vi "Control_DAQ.vi"(7 "Transfer Function":T5={"Transfer Function"={"Numerator"=[1.0], "Denominator"=[-0.9, 1.0]}, "Limit Cluster"={"Upper Limit"=0.0, "Lower Limit"=0.0}}, 8 "error in":errorcluster, 9 "Time":dbl format="%#_13g", 11 "Inputs":T2={"File Name"="", "Force (Hz)"=0.0, "Camera (Hz)"=0.0, "Systole (V)"=0.0, "Diastole (V)"=0.0, "T (sec)"=0.0, "Delay (sec)"=0.0, "Setpoint Function"=enum."Incremental PWM Step", "Max Diam (mm)"=0.0, "DAQmx Servo Task"="MyPulseOutputTask", "Force Sensor Channel"="Dev2/ai7", "DAQmx LED Task"="MyDigitalOutTask", "Camera Selector"="cam5", "FS Task Out"="", "Servo Task Out"="", "LED Task Out"="", "Camera Session Out"="", "Color Pane"=0} {"Color Pane" items=["Blue", "Red", "Green", "Saturation", "Value", "Intensity", "Luminance", "Hue", ""]}) -> (0 "error out":errorcluster, 2 "Force cluster":T1, 3 "Inputs Out":T2={"File Name"="", "Force (Hz)"=0.0, "Camera (Hz)"=0.0, "Systole (V)"=0.0, "Diastole (V)"=0.0, "T (sec)"=0.0, "Delay (sec)"=0.0, "Setpoint Function"=enum."Incremental PWM Step", "Max Diam (mm)"=0.0, "DAQmx Servo Task"="MyPulseOutputTask", "Force Sensor Channel"="Dev2/ai7", "DAQmx LED Task"="MyDigitalOutTask", "Camera Selector"="cam5", "FS Task Out"="", "Servo Task Out"="", "LED Task Out"="", "Camera Session Out"="", "Color Pane"=0} {"Color Pane" items=["Blue", "Red", "Green", "Saturation", "Value", "Intensity", "Luminance", "Hue", ""]}, 6 "Time Exceeded?":bool)   [LabVIEW 2020]
uses:
  Controls/Inputs.ctl
  Controls/Serpoint.ctl
  <vilib>/userDefined/High Color/IMAQdx.ctl
  Controls/controlspec.ctl
  Controls/ForceCluster.ctl
  <vilib>/DAQmx/read.llb/DAQmx Read (Analog 1D DBL 1Chan NSamp).vi
  <vilib>/DAQmx/write.llb/DAQmx Write (Digital Bool 1Line 1Point).vi
  <vilib>/DAQmx/write.llb/DAQmx Write (Counter Frequency 1Chan 1Samp).vi
  <vilib>/DAQmx/miscellaneous.llb/DAQmx Fill In Error Info.vi
panel:
  in  "Slope":dbl format="%#_13g"
  # "Test Variables:"
  # "Sampling Frequencies:"
  # "Test Variables:"
  # "Sampling Frequencies:"
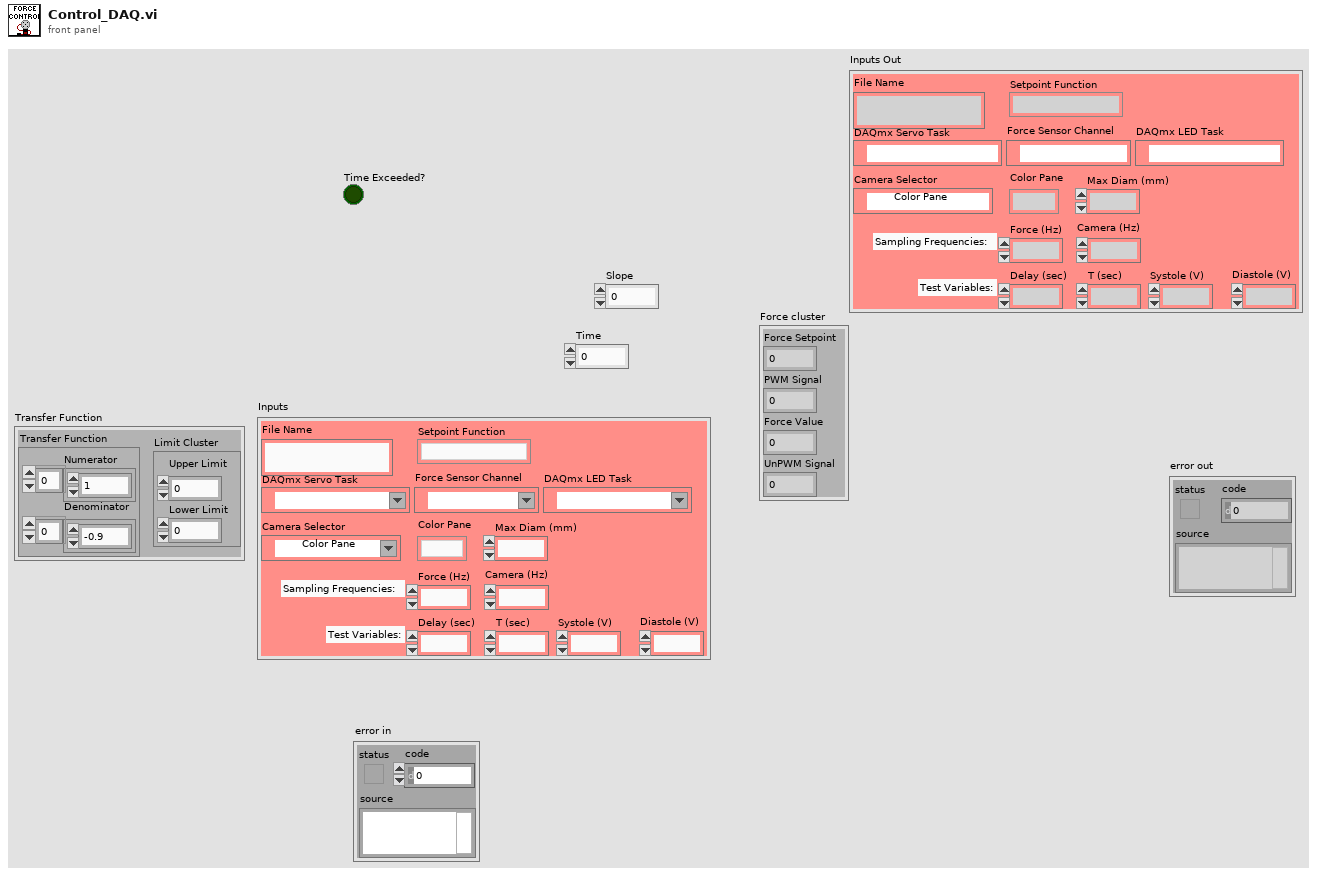
[diagram p1: front panel]
types:
  T1 = typedef "ForceCluster.ctl" = cluster{"Force Setpoint":dbl, "PWM Signal":dbl, "Force Value":dbl, "UnPWM Signal":dbl}
  T2 = typedef "Inputs.ctl" = cluster{"File Name":string, "Force (Hz)":dbl, "Camera (Hz)":dbl, "Systole (V)":dbl, "Diastole (V)":dbl, "T (sec)":dbl, "Delay (sec)":dbl, "Setpoint Function":T3, "Max Diam (mm)":dbl, "DAQmx Servo Task":refnum<k21>, "Force Sensor Channel":tag, "DAQmx LED Task":refnum<k21>, "Camera Selector":T4, "FS Task Out":refnum<k21>, "Servo Task Out":refnum<k21>, "LED Task Out":refnum<k21>, "Camera Session Out":T4, "Color Pane":i32}
  T3 = typedef "Serpoint.ctl" = enum16{"Incremental PWM Step", "PWM Step", "Ramp", "Sinusoidal", "Blood-Pressure"}
  T4 = typedef "IMAQdx.ctl" = refnum<k21>
  T5 = typedef "controlspec.ctl" = cluster{"Transfer Function":cluster{"Numerator":dbl[], "Denominator":dbl[]}, "Limit Cluster":cluster{"Upper Limit":dbl, "Lower Limit":dbl}}
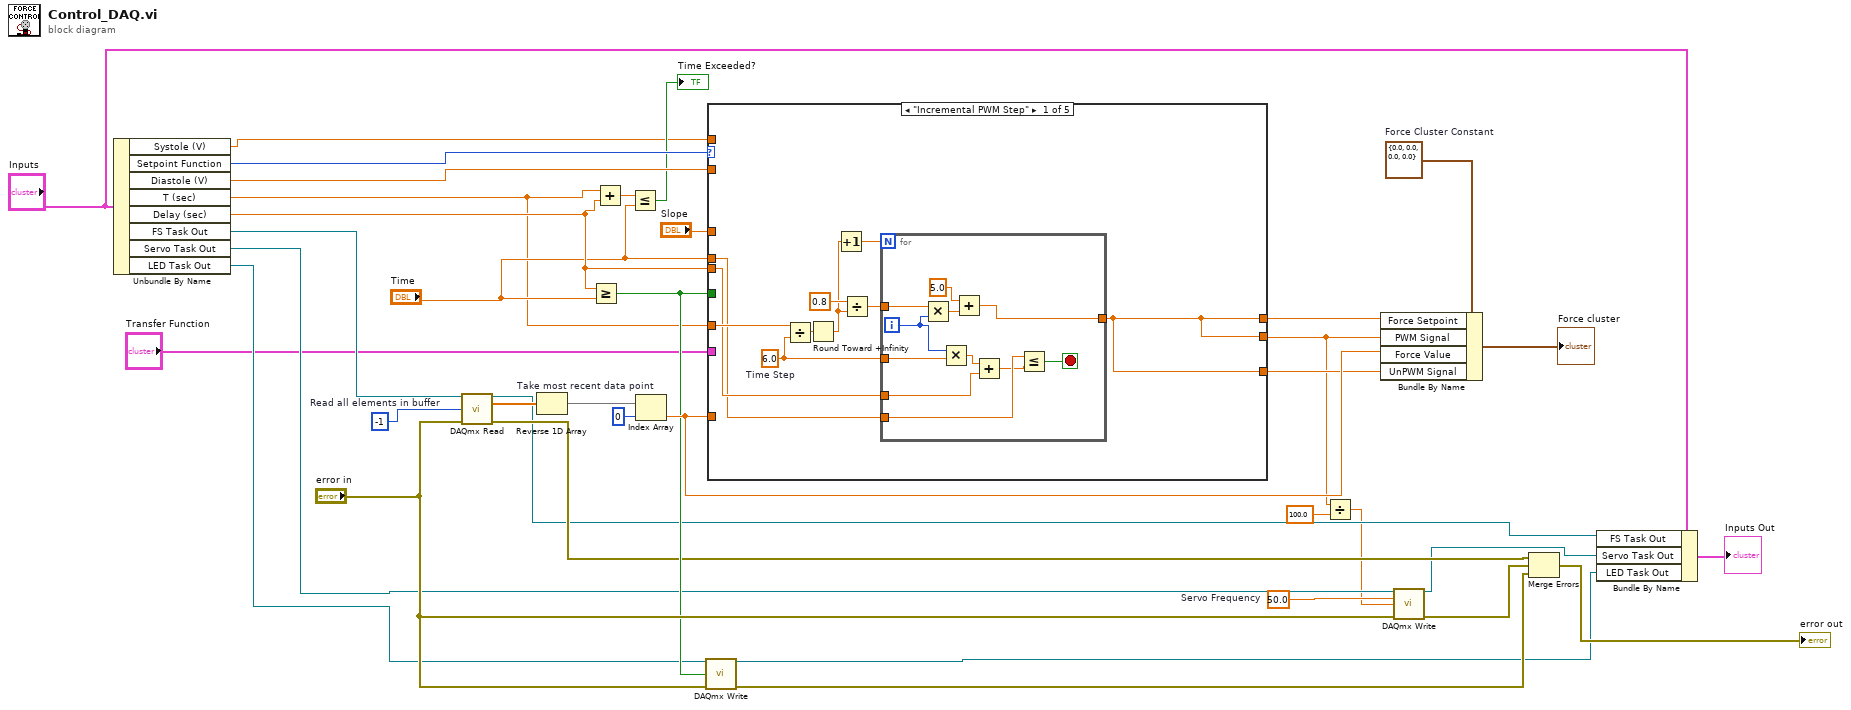
[diagram p0: block diagram]
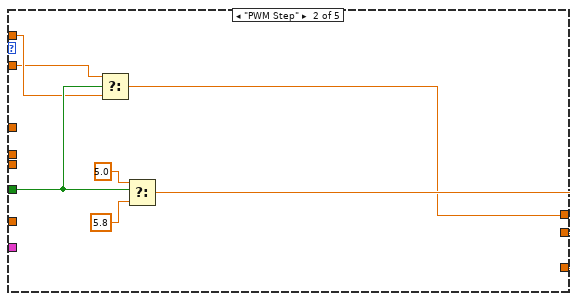
[diagram p2: hidden frame]
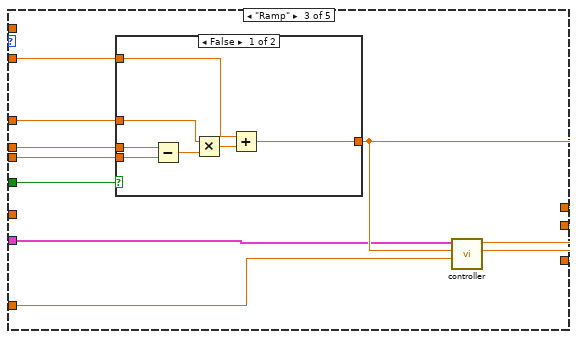
[diagram p3: hidden frame]
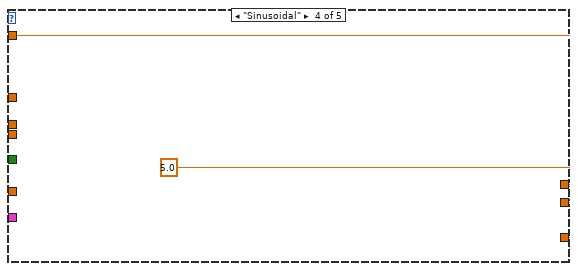
[diagram p5: hidden frame]
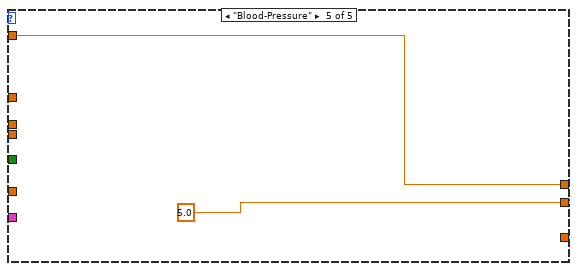
[diagram p6: hidden frame]
diagram:
  w17 = 50.0  # Servo Frequency
  w26 = T1 {"Force Setpoint"=0.0, "PWM Signal"=0.0, "Force Value"=0.0, "UnPWM Signal"=0.0}  # Force Cluster Constant
  w30 = -1  # Read all elements in buffer
  n1 = Unbundle By Name("Inputs") -> ("Systole (V)"=w2:dbl, "Setpoint Function"=w37:T3, "Diastole (V)"=w34:dbl, "T (sec)"=w1:dbl, "Delay (sec)"=w36:dbl, "FS Task Out"=w13:refnum<k21>, "Servo Task Out"=w14:refnum<k21>, "LED Task Out"=w15:refnum<k21>)
  n2 = call-poly <vilib>:"DAQmx Read.vi"("task/channels in"=w13, "number of samples per channel"=w30, "error in"="error in") -> ("task out"=w12:refnum<k21>, "data"=w29:dbl[], "error out"=w20:errorcluster)  [unwired: 10 in]
  n3 = Reverse 1D Array(array=w29) -> (reversed array=w28:dbl[])
  n4 = Greater Or Equal?(x=w36, y="Time") -> (x >= y?=w22:bool)
  n5 = Add(x=w1, y=w36) -> (x+y=w33:dbl)
  n6 = Less Or Equal?(x=w33, y="Time") -> (x <= y?=→"Time Exceeded?":bool)
  n7 = Index Array "Take most recent data point"(array=w28, index=0) -> (element=w24:dbl)
  n8 = call-poly <vilib>:"DAQmx Write.vi"("task/channels in"=w15, "data"=w22, "error in"="error in") -> ("task out"=w10:refnum<k21>, "error out"=w18:errorcluster)  [unwired: 10 in, 1 out]
  n9 = case shown="\"Incremental PWM Step\"" w37 {
    tunnel: w22 -> [_ w62 w75 _ _]
    tunnel: w36 -> [w44 _ w74 _ _]
    tunnel: "Time" -> [w42 _ w73 _ _]
    tunnel: "Slope" -> [_ _ w72 _ _]
    tunnel: w34 -> [_ w60 w71 w84 w86]
    tunnel: w24 -> [_ _ w68 _ _]
    tunnel: [w38 w63 w67 w85 w87] -> w6
    tunnel: [w38 w59 w69 w84 w86] -> w25
    tunnel: [w38 w63 w70 w85 w87] -> w16
    tunnel: "Transfer Function" -> [_ _ w66 _ _]
    tunnel: w2 -> [_ w61 _ _ _]
    tunnel: w1 -> [w47 _ _ _ _]
    frame "Incremental PWM Step" {
      w45 = 6.0  # Time Step
      n10 = Divide(x=w47, y=w45) -> (x/y=w46:dbl)
      n11 = Round Toward +Infinity(x=w46) -> (ceil(x): smallest int >= x=w41:dbl)
      n12 = Increment(x=w41) -> (x+1=w40:dbl)
      n13 = Divide(x=0.8, y=w41) -> (x/y=w39:dbl)
      n14 = for {
        N: w40 -> [_]
        tunnel: w45 -> [w53]
        tunnel: w44 -> [w57]
        tunnel: w42 -> [w56]
        tunnel: [w49] -> w38
        tunnel: w39 -> [w48]
        i -> [w50]
        stop <- w54 stop-if-true
        n15 = Multiply(x=w48, y=w50) -> (x*y=w51:dbl)
        n16 = Multiply(x=w50, y=w53) -> (x*y=w58:dbl)
        n17 = Add(x=5.0 ("Output"), y=w51) -> (x+y=w49:dbl)
        n18 = Add(x=w58, y=w57) -> (x+y=w55:dbl)
        n19 = Less Or Equal?(x=w56, y=w55) -> (x <= y?=w54:bool)
      }
    }
    frame "PWM Step" {
      n20 = Select(t=w60, s=w62, f=w61) -> (s? t:f=w59:dbl)
      n21 = Select(t=5.0 ("Output"), s=w62, f=5.8 ("Output")) -> (s? t:f=w63:dbl)
    }
    frame "Ramp" {
      n22 = case shown="False" w75 {
        tunnel: w74 -> [w82 _]
        tunnel: w73 -> [w81 _]
        tunnel: w72 -> [w77 _]
        tunnel: w71 -> [w79 w83]
        tunnel: [w76 w83] -> w69
        frame False {
          n23 = Subtract(x=w81, y=w82) -> (x-y=w78:dbl)
          n24 = Multiply(x=w77, y=w78) -> (x*y=w80:dbl)
          n25 = Add(x=w79, y=w80) -> (x+y=w76:dbl)
        }
        frame True {
        }
      }
      n26 = call "controller.vi"("FS Data"=w68, "Setpoint"=w69, "Cluster"=w66) -> ("Uncoerced Output"=w70:dbl, "Output"=w67:dbl)  [unwired: 6 in, 1 out]
    }
    frame "Sinusoidal" {
      w85 = 5.0
    }
    frame "Blood-Pressure" {
      w87 = 5.0
    }
  }
  n27 = Divide(x=w6, y=100.0) -> (x/y=w5:dbl)
  n28 = Bundle By Name(cluster=w26, "Force Setpoint"=w25, "PWM Signal"=w6, "Force Value"=w24, "UnPWM Signal"=w16) -> (→"Force cluster":T1)
  n29 = call-poly <vilib>:"DAQmx Write.vi"("task/channels in"=w14, "frequency"=w17, "duty cycle"=w5, "error in"="error in") -> ("task out"=w11:refnum<k21>, "error out"=w19:errorcluster)  [unwired: 9 in, 1 out]
  n30 = Merge Errors(w20, w19, w18) -> (→"error out":errorcluster)
  n31 = Bundle By Name(cluster="Inputs", "FS Task Out"=w12, "Servo Task Out"=w11, "LED Task Out"=w10) -> (→"Inputs Out":T2)
